vi "Teleop.vi"(10 "Match Info":T4={"Autonomous Elapsed Seconds"=0.0, "TeleOp Elapsed Seconds"=0.0, "Disabled Elapsed Seconds"=0.0, "Visited Autonomous"=FALSE, "Visited TeleOp"=FALSE, "Visited Disabled"=FALSE, "Autonomous Settings"={"Autonomous Style"=enum."Independent", "VI Refnum"=refnum}}, 11 "Call Context":T5) -> ()   [LabVIEW 2013]
doc: "This VI is called for each TeleOp packet received from the DS where the robot is not disabled. It is often used to read from the joysticks and update I/O or to update setpoints for timed control loops. It should complete and return within 20 milliseconds or it may miss DS packets."
uses:
  <vilib>/Rock Robotics/WPI/DriverStation/WPI_DriverStationDerivedRobotMode.ctl
  <vilib>/Rock Robotics/WPI/DriverStation/WPI_DriverStationMatch Info.ctl
  <vilib>/Rock Robotics/WPI/Solenoid/WPI_SolenoidValue.ctl
  <vilib>/Rock Robotics/WPI/Relay/WPI_RelayValue.ctl
  Robot Global Data.vi
  <vilib>/Rock Robotics/Network Tables/SD Read Number.vi
  <vilib>/Rock Robotics/WPI/Solenoid/WPI_SolenoidGetEnum.vi
  <vilib>/Rock Robotics/WPI/Compressor/WPI_CompressorGetSetRefNum.vi
  <vilib>/Rock Robotics/WPI/Solenoid/WPI_SolenoidSetEnum.vi
  <vilib>/Rock Robotics/WPI/Joystick/WPI_JoystickGetSetRefNum.vi
  <vilib>/Rock Robotics/WPI/RobotDrive/WPI_RobotDriveGetSetRefNum.vi
panel:
  in  "Grabber Timer":dbl
  in  "GrabberCurrentTarget":dbl
  in  "HasGrabberBeenReset":bool
  in  "ToughBoxEncoderTopPosition":dbl
  in  "Current Grabber Status":T1(ring)
  out "Waveform Chart 2":dbl(graph)
  in  "Run Grabber PID 2":bool
  out "Reed Switch 2":bool
  out "Reed Switch 1":bool
  out "Top Limit Tripped":bool
  out "Micro Switch":bool
  out "Bottom Limit Tripped":bool
  out "Axis Value  6":dbl
  out "Axis Value 5":dbl
  out "Axis Value 4":dbl
  in  "Grabber Axis Value":T2(ring)
  in  "Current Shooter Status":T3(ring)
  out "Waveform Chart":dbl(graph)
  out "Mechanism Moving Up":bool
  out "Mechanism Moving Down":bool
  out "Time Since Button Pressed":dbl
  in  "Manual Override Activated":bool
  in  "Button 2 Pressed":bool
  in  "Firing Pin Forward":bool
  in  "Mechanism Piston Forward":bool
  in  "Tick Taken":bool
  out "Time at Gather":dbl
  out "Timer for firing mech":dbl
  in  "Mechanism Status":string
types:
  T1 = enum16{"Resetting", "Going Up", "Going Up Slow", "In Shooting Position", "Going Down", "Going Down Slow", "In Loading Position"}
  T2 = enum16{"Less Than Zero", "Greater Than Zero", "Equal To Zero"}
  T3 = enum16{"Retracting", "Firing", "Ready to fire", "Pulling back", "Just fired"}
  T4 = typedef "WPI_DriverStationMatch Info.ctl" = cluster{"Autonomous Elapsed Seconds":dbl, "TeleOp Elapsed Seconds":dbl, "Disabled Elapsed Seconds":dbl, "Visited Autonomous":bool, "Visited TeleOp":bool, "Visited Disabled":bool, "Autonomous Settings":cluster{"Autonomous Style":enum16{"Iterative", "Independent"}, "VI Refnum":refnum<vi>}}
  T5 = typedef "WPI_DriverStationDerivedRobotMode.ctl" = enum16{"Init", "Execute", "Stop"}
  T6 = typedef "WPI_SolenoidValue.ctl" = enum16{"Off", "On", "Forward", "Reverse"}
  T7 = enum16{"Resetting", "Going Up", "Going Up Slow", "In Shooting Position", "Going Down", "Going Down Slow", "In Loading Position", ""}
  T8 = typedef "WPI_DigitalInputDevRef.ctl" = cluster{"DevStatus":errorcluster, "DIO Channel":T9, "Digital Module":T10}
  T9 = typedef "FPGA_DIOChannel.ctl" = enum8{"DIO 1", "DIO 2", "DIO 3", "DIO 4", "DIO 5", "DIO 6", "DIO 7", "DIO 8", "DIO 9", "DIO 10", "DIO 11", "DIO 12", "DIO 13", "DIO 14", "Invalid"}
  T10 = typedef "FPGA_TypedefDigitalModule.ctl" = enum16{"Digital Module 1", "Digital Module 2"}
  T11 = typedef "WPI_MotorControlDeviceRef.ctl" = cluster{"DeviceStatus":errorcluster, "Type":enum16{"PWM", "CAN"}, "PWM":cluster{"Digital Module":T10, "PWM Channel":T12, "DeadBand":T13}, "CAN":cluster{"Device Number":u8, "Control Mode":T14, "Semaphore":T15, "Max Vout":dbl}, "Invert":bool, "TransformRef":T16, "InvTransformRef":T16}
  T12 = typedef "FPGA_DIOPWMChannel.ctl" = enum8{"PWM 1", "PWM 2", "PWM 3", "PWM 4", "PWM 5", "PWM 6", "PWM 7", "PWM 8", "PWM 9", "PWM 10", "Invalid"}
  T13 = typedef "WPI_PWMDeadband.ctl" = cluster{"Name":string, "maxPositivePwm":i32, "minPositivePwm":i32, "centerPwm":i32, "maxNegativePwm":i32, "minNegativePwm":i32, "angularRange":u16}
  T14 = typedef "WPI_CANJaguar_ControlMode.ctl" = enum8{"Percent VBus", "Current", "Speed", "Position", "Voltage"}
  T15 = typedef "Semaphore RefNum" = refnum<k1>
  T16 = typedef "WPI_PWMTransform_ConPane.ctl" = refnum<vi>
  T17 = typedef "WPI_SolenoidDevRef.ctl" = cluster{"DevStatus":errorcluster, "Solenoid Module":T18, "Forward Solenoid Channel":T19, "Reverse Solenoid Channel":T19}
  T18 = typedef "FPGA_TypedefSolenoidModule.ctl" = enum16{"Solenoid Module 1", "Solenoid Module 2"}
  T19 = typedef "WPI_SolenoidChannel.ctl" = enum8{"Solenoid 1", "Solenoid 2", "Solenoid 3", "Solenoid 4", "Solenoid 5", "Solenoid 6", "Solenoid 7", "Solenoid 8", "Invalid"}
  T20 = typedef "WPI_JoystickDevRef.ctl" = cluster{"Device":T21}
  T21 = typedef "WPI_JoystickDeviceEnum.ctl" = enum16{"USB 1", "USB 2", "USB 3", "USB 4", "Kinect 1", "Kinect 2"}
  T22 = typedef "WPI_JoystickButtonState.ctl" = cluster{"Button 1":bool, "Button 2":bool, "Button 3":bool, "Button 4":bool, "Button 5":bool, "Button 6":bool, "Button 7":bool, "Button 8":bool, "Button 9":bool, "Button 10":bool, "Button 11":bool, "Button 12":bool}
  T23 = typedef "WPI_EncoderDevRef.ctl" = cluster{"DevStatus":errorcluster, "EncoderIndex":T24, "CounterIndex":T25, "DistancePerCount":dbl, "Decoding Type":T26}
  T24 = typedef "FPGA_EncoderIdx.ctl" = enum8{"Enc 0", "Enc 1", "Enc 2", "Enc 3", "Invalid"}
  T25 = typedef "FPGA_CounterCtrSystemIndex.ctl" = enum8{"Ctr 0", "Ctr 1", "Ctr 2", "Ctr 3", "Ctr 4", "Ctr 5", "Ctr 6", "Ctr 7", "Invalid"}
  T26 = typedef "WPI_EncoderType.ctl" = enum16{"1x", "2x", "4x"}
  T27 = typedef "WPI_RelayDevRef.ctl" = cluster{"DevStatus":errorcluster, "Relay Channel":T28, "Digital Module":T10, "Relay Direction":T29}
  T28 = typedef "FPGA_DIORelayChannel.ctl" = enum8{"Relay 1", "Relay 2", "Relay 3", "Relay 4", "Relay 5", "Relay 6", "Relay 7", "Relay 8", "Invalid"}
  T29 = typedef "WPI_RelayDirection.ctl" = enum16{"Both directions", "Forward only", "Reverse only"}
  T30 = typedef "WPI_CompressorDevRef.ctl" = cluster{"DevStatus":errorcluster, "DigitalInputDevRef":T8, "RelayDevRef":T27}
  T31 = typedef "WPI_RelayValue.ctl" = enum16{"Off", "On", "Forward", "Reverse"}
  T32 = typedef "WPI_AnalogChannelDevRef.ctl" = cluster{"DevStatus":errorcluster, "Analog Module":T33, "Analog Channel":T34}
  T33 = typedef "FPGA_TypedefAnalogModule.ctl" = enum16{"Analog Module 1", "Analog Module 2"}
  T34 = typedef "FPGA_AIChannel.ctl" = enum8{"AI 1", "AI 2", "AI 3", "AI 4", "AI 5", "AI 6", "AI 7", "AI 8", "Invalid"}
  T35 = typedef "WPI_ServoDeviceRef.ctl" = cluster{"DeviceStatus":errorcluster, "Digital Module":T10, "PWM Channel":T12, "DeadBand":T13}
  T36 = cluster{"axis 1 (x)":dbl, "axis 2 (y)":dbl, "axis 3 (throttle)":dbl, "axis 4":dbl, "axis 5":dbl, "axis 6":dbl}
  T37 = typedef "WPI_RobotDriveDevRef.ctl" = cluster{"DevStatus":errorcluster, "Motors[]":T11[], "Square Inputs":bool, "Max Output":dbl, "Isochronous":bool}
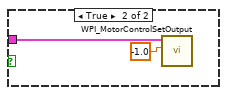
[diagram p3: hidden frame]
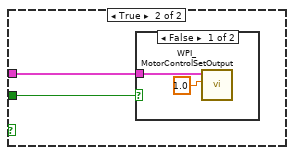
[diagram p4: hidden frame]
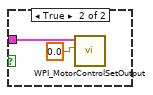
[diagram p5: hidden frame]
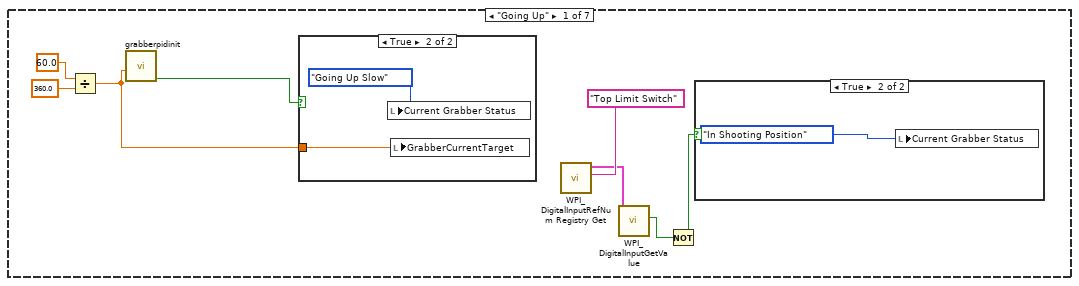
[diagram p7: hidden frame]
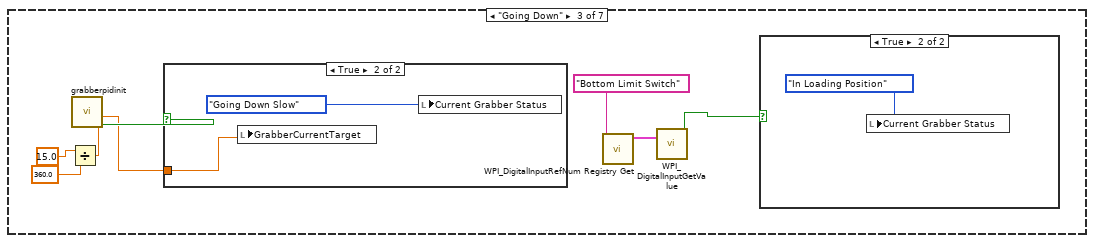
[diagram p11: hidden frame]
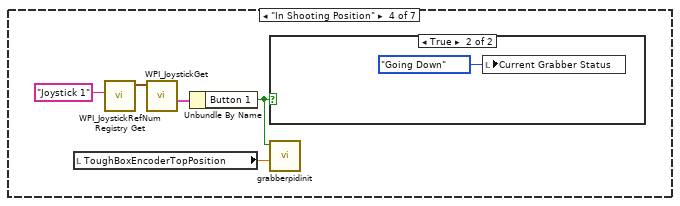
[diagram p14: hidden frame]
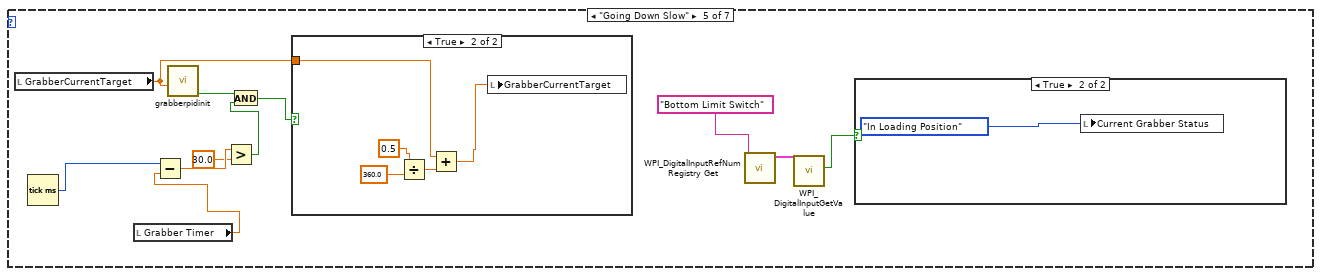
[diagram p16: hidden frame]
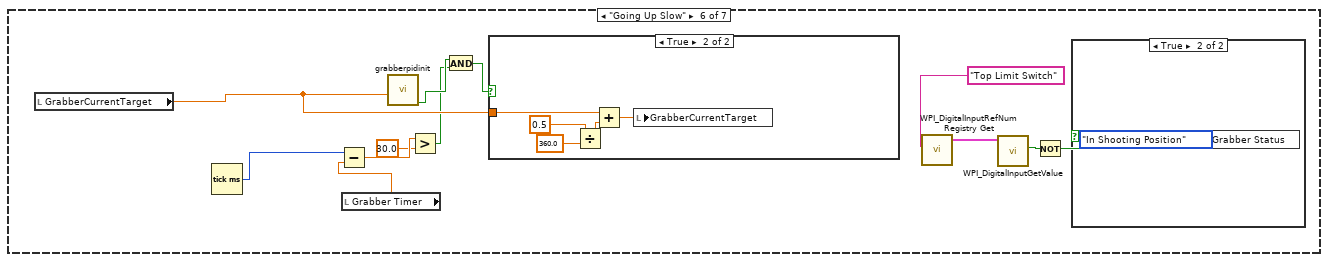
[diagram p19: hidden frame]
diagram:
  (unwired) "Below code is for running the Raising/Lowering motors"
  (unwired) "This code sets the toggle rate used by the Periodic Tasks VI.  For teleop mode we flash the USER1 LED on the cRIO at a fast rate.  Look at the Periodic Tasks VI to see how this global value is used."
  (unwired) "This VI is called each time a TeleOp DS packet is received.  Use it to respond to new joystick or Driver Station values.\n\nCommon tasks include reading the joysticks and updating motors, and updating setpoints for periodic loops.\n\nYou can open I/O on the FIRST Call, or in the Begin.vi."
  # "one encoder"
  # "Check me!"
  # "If no buttons pressed - 0\nIf left pressed = 7\nIf right pressed = -7\nIf both = 0"
  # "Publish the Robot Drive Motor\nvalues to the dashboard"
  # "Publish the joystick data the\nrobot sees to the dashboard"
  # "Each time we enter, report that\nwe are running teleop"
  # "Use to differentiate between\nFirst, Last, and Intermediate calls"
  # "Read Joystick X and Y values and update motor values"
  n1 = call <vilib>:"SD Read Boolean.vi"("Name"="Manual Mechanism Override") -> ("Boolean"=w7:bool)  [unwired: 8 in, 2 out]
  n2 = Not(x=w7) -> (.not. x?=w8:bool)
  n3 = case shown="True" w8 {
    frame False {
    }
    frame True {
      n4 = local read "Current Grabber Status"() -> (w131:T1)
      n5 = case shown="\"In Loading Position\"" w131 {
        frame "Going Up" {
          n6 = Divide(x=60.0 ("setpoint"), y=360.0) -> (x/y=w132:dbl)
          n7 = call "grabberpidinit.vi"("setpoint"=w132) -> ("Done? 2"=w139:bool)  [unwired: 10 in]
          n8 = case shown="True" w139 {
            tunnel: w132 -> [_ w141]
            frame False {
            }
            frame True {
              n9 = local write "Current Grabber Status"(T1."Going Up Slow" ("Current Grabber Status")) -> ()
              n10 = local write "GrabberCurrentTarget"(w141) -> ()
            }
          }
          n11 = call <vilib>:"WPI_DigitalInputRefNum Registry Get.vi"("refnum name"="Top Limit Switch") -> ("DigitalInputDevRef"=w137:T8)  [unwired: 9 in, 1 out]
          n12 = call <vilib>:"WPI_DigitalInputGetValue.vi"("DigitalInputDevRef"=w137) -> ("Value"=w136:bool)  [unwired: 8 in, 2 out]
          n13 = Not(x=w136) -> (.not. x?=w135:bool)
          n14 = case shown="True" w135 {
            frame False {
            }
            frame True {
              n15 = local write "Current Grabber Status"(T1."In Shooting Position" ("Current Grabber Status")) -> ()
            }
          }
        }
        frame "In Loading Position" {
          # "Change to the UltraSonic Sensor\nwhen possible"
          n16 = call "grabberpidinit.vi"("setpoint"=0.0) -> ("Done? 2"=w143:bool)  [unwired: 10 in]
          n17 = call <vilib>:"WPI_MotorControlRefNum Registry Get.vi"("refnum name"="Snowblower") -> ("MotorControlDevRef"=w155:T11)  [unwired: 9 in, 1 out]
          n18 = call <vilib>:"WPI_MotorControlSetOutput.vi"("Output"=-1.0, "MotorControlDevRef"=w155) -> ()  [unwired: 7 in, 3 out]
          n19 = call <vilib>:"WPI_SolenoidRefNum Registry Get.vi"("refnum name"="Grabber Pistons Solenoid") -> ("error out"=w152:errorcluster, "SolenoidDevRef"=w151:T17)  [unwired: 9 in]
          n20 = call-poly <vilib>:"WPI_SolenoidSet.vi"("error in (no error)"=w152, "Value"=WPI_SolenoidValue."Reverse", "SolenoidDevRef"=w151) -> ()  [unwired: 7 in, 2 out]
          n21 = call <vilib>:"WPI_JoystickRefNum Registry Get.vi"("refnum name"="Joystick 1") -> ("JoystickDevRef"=w147:T20)  [unwired: 1 in, 9 out]
          n22 = call <vilib>:"WPI_JoystickGet.vi"("JoystickDevRef"=w147) -> ("Buttons"=w146:T22)  [unwired: 1 in, 5 out]
          n23 = Unbundle By Name(w146) -> ("Button 4"=w144:bool)
          n24 = And(x=w143, y=w144) -> (x .and. y?=w145:bool)
          n25 = case shown="True" w145 {
            frame False {
            }
            frame True {
              n26 = local write "Current Grabber Status"(T1."Going Up" ("Current Grabber Status")) -> ()
            }
          }
        }
        frame "Going Down" {
          n27 = Divide(x=15.0, y=360.0) -> (x/y=w158:dbl)
          n28 = call "grabberpidinit.vi"("setpoint"=w158) -> ("Done? 2"=w164:bool)  [unwired: 10 in]
          n29 = case shown="True" w164 {
            tunnel: w158 -> [_ w166]
            frame False {
            }
            frame True {
              n30 = local write "GrabberCurrentTarget"(w166) -> ()
              n31 = local write "Current Grabber Status"(T1."Going Down Slow" ("Current Grabber Status")) -> ()
            }
          }
          n32 = call <vilib>:"WPI_DigitalInputRefNum Registry Get.vi"("refnum name"="Bottom Limit Switch") -> ("DigitalInputDevRef"=w162:T8)  [unwired: 9 in, 1 out]
          n33 = call <vilib>:"WPI_DigitalInputGetValue.vi"("DigitalInputDevRef"=w162) -> ("Value"=w161:bool)  [unwired: 8 in, 2 out]
          n34 = case shown="True" w161 {
            frame False {
            }
            frame True {
              n35 = local write "Current Grabber Status"(T1."In Loading Position" ("Current Grabber Status")) -> ()
            }
          }
        }
        frame "In Shooting Position" {
          n36 = local read "ToughBoxEncoderTopPosition"() -> (w169:dbl)
          n37 = call <vilib>:"WPI_JoystickRefNum Registry Get.vi"("refnum name"="Joystick 1") -> ("JoystickDevRef"=w171:T20)  [unwired: 1 in, 9 out]
          n38 = call <vilib>:"WPI_JoystickGet.vi"("JoystickDevRef"=w171) -> ("Buttons"=w170:T22)  [unwired: 1 in, 5 out]
          n39 = Unbundle By Name(w170) -> ("Button 1"=w168:bool)
          n40 = case shown="True" w168 {
            frame False {
            }
            frame True {
              n41 = local write "Current Grabber Status"(T7."Going Down" ("Current Grabber Status")) -> ()
            }
          }
          n42 = call "grabberpidinit.vi"("setpoint"=w169, "reinitialize? (F) 2"=w168) -> ()  [unwired: 9 in, 1 out]
        }
        frame "Going Down Slow" {
          n43 = local read "GrabberCurrentTarget"() -> (w174:dbl)
          n44 = Tick Count (ms)() -> (millisecond timer value=w184:u32)
          n45 = local read "Grabber Timer"() -> (w181:dbl)
          n46 = Subtract(x=w184, y=w181) -> (x-y=w183:dbl)
          n47 = call "grabberpidinit.vi"("setpoint"=w174) -> ("Done? 2"=w180:bool)  [unwired: 10 in]
          n48 = Greater?(x=w183, y=30.0) -> (0:w179:bool)
          n49 = And(x=w180, y=w179) -> (x .and. y?=w178:bool)
          n50 = case shown="True" w178 {
            tunnel: w174 -> [_ w187]
            frame False {
            }
            frame True {
              n51 = Divide(x=0.5, y=360.0) -> (x/y=w188:dbl)
              n52 = Add(x=w187, y=w188) -> (x+y=w186:dbl)
              n53 = local write "GrabberCurrentTarget"(w186) -> ()
            }
          }
          n54 = call <vilib>:"WPI_DigitalInputRefNum Registry Get.vi"("refnum name"="Bottom Limit Switch") -> ("DigitalInputDevRef"=w176:T8)  [unwired: 9 in, 1 out]
          n55 = call <vilib>:"WPI_DigitalInputGetValue.vi"("DigitalInputDevRef"=w176) -> ("Value"=w175:bool)  [unwired: 8 in, 2 out]
          n56 = case shown="True" w175 {
            frame False {
            }
            frame True {
              n57 = local write "Current Grabber Status"(T1."In Loading Position" ("Current Grabber Status")) -> ()
            }
          }
        }
        frame "Going Up Slow" {
          n58 = local read "GrabberCurrentTarget"() -> (w202:dbl)
          n59 = Tick Count (ms)() -> (millisecond timer value=w201:u32)
          n60 = local read "Grabber Timer"() -> (w200:dbl)
          n61 = Subtract(x=w201, y=w200) -> (x-y=w199:dbl)
          n62 = call "grabberpidinit.vi"("setpoint"=w202) -> ("Done? 2"=w197:bool)  [unwired: 10 in]
          n63 = Greater?(x=w199, y=30.0) -> (0:w196:bool)
          n64 = And(x=w197, y=w196) -> (x .and. y?=w195:bool)
          n65 = case shown="True" w195 {
            tunnel: w202 -> [_ w207]
            frame False {
            }
            frame True {
              n66 = Divide(x=0.5 ("y"), y=360.0) -> (x/y=w204:dbl)
              n67 = Add(x=w207, y=w204) -> (x+y=w208:dbl)
              n68 = local write "GrabberCurrentTarget"(w208) -> ()
            }
          }
          n69 = call <vilib>:"WPI_DigitalInputRefNum Registry Get.vi"("refnum name"="Top Limit Switch") -> ("DigitalInputDevRef"=w192:T8)  [unwired: 9 in, 1 out]
          n70 = call <vilib>:"WPI_DigitalInputGetValue.vi"("DigitalInputDevRef"=w192) -> ("Value"=w194:bool)  [unwired: 8 in, 2 out]
          n71 = Not(x=w194) -> (.not. x?=w193:bool)
          n72 = case shown="True" w193 {
            frame False {
            }
            frame True {
              n73 = local write "Current Grabber Status"(T1."In Shooting Position" ("Current Grabber Status")) -> ()
            }
          }
        }
        frame "Resetting", Default {
          n74 = local read "GrabberCurrentTarget"() -> (w221:dbl)
          n75 = call <vilib>:"WPI_DigitalInputRefNum Registry Get.vi"("refnum name"="Bottom Limit Switch") -> ("DigitalInputDevRef"=w211:T8)  [unwired: 9 in, 1 out]
          n76 = Equal?(x=w221, y=0.0) -> (x = y?=w220:bool)
          n77 = call <vilib>:"WPI_DigitalInputGetValue.vi"("DigitalInputDevRef"=w211) -> ("Value"=w209:bool)  [unwired: 8 in, 2 out]
          n78 = case shown="True" w220 {
            tunnel: [w233 w234] -> w219
            tunnel: w221 -> [w233 _]
            frame False {
            }
            frame True {
              # "one encoder"
              n79 = call <vilib>:"WPI_EncoderRefNum Registry Get.vi"("refnum name"="Tough Box Encoder") -> ("error out"=w237:errorcluster, "EncoderDevRef"=w236:T23)  [unwired: 9 in]
              n80 = call <vilib>:"WPI_EncoderGet.vi"("error in (no error)"=w237, "EncoderDevRef"=w236) -> ("Distance"=w234:dbl)  [unwired: 4 in, 5 out]
              n81 = local write "GrabberCurrentTarget"(w234) -> ()
            }
          }
          n82 = case shown="True" w209 {
            frame False {
            }
            frame True {
              n83 = call <vilib>:"WPI_EncoderRefNum Registry Get.vi"("refnum name"="Tough Box Encoder") -> ("error out"=w225:errorcluster, "EncoderDevRef"=w224:T23)  [unwired: 9 in]
              n84 = local write "Current Grabber Status"(T7."In Loading Position" ("Current Grabber Status")) -> ()
              n85 = call <vilib>:"WPI_EncoderReset.vi"("error in (no error)"=w225, "EncoderDevRef"=w224) -> ()  [unwired: 8 in, 2 out]
            }
          }
          n86 = local read "Grabber Timer"() -> (w217:dbl)
          n87 = Tick Count (ms)() -> (millisecond timer value=w218:u32)
          n88 = Subtract(x=w218, y=w217) -> (x-y=w216:dbl)
          n89 = call "grabberpidinit.vi"("setpoint"=w219, "reinitialize? (F) 2"=w209) -> ("Done? 2"=w212:bool)  [unwired: 9 in]
          n90 = Greater?(x=w216, y=30.0) -> (0:w213:bool)
          n91 = And(x=w212, y=w213) -> (x .and. y?=w214:bool)
          n92 = case shown="True" w214 {
            tunnel: w219 -> [_ w229]
            frame False {
            }
            frame True {
              n93 = Tick Count (ms)() -> (millisecond timer value=w227:u32)
              n94 = Divide(x=0.5, y=360.0) -> (x/y=w232:dbl)
              n95 = Subtract(x=w229, y=w232) -> (x-y=w228:dbl)
              n96 = local write "Grabber Timer"(w227) -> ()
              n97 = local write "GrabberCurrentTarget"(w228) -> ()
            }
          }
        }
      }
    }
  }
  n98 = local write "Mechanism Piston Forward"(FALSE) -> ()
  n99 = local write "Firing Pin Forward"(FALSE) -> ()
  n100 = call <vilib>:"WPI_DriverStationReport Robot Code State.vi"("TeleOp"=TRUE ("Autonomous")) -> ()  [unwired: 10 in, 1 out]
  n101 = global write "Robot Global Data.vi" "LED toggle rate (ms)"(u32 100 ("LED ms toggle rate")) -> ()
  n102 = call <vilib>:"WPI_JoystickRefNum Registry Get.vi"("refnum name"="Joystick 1") -> ("JoystickDevRef"=w109:T20)  [unwired: 1 in, 9 out]
  n103 = Unbundle By Name("Match Info") -> ()  [unwired: 1 out]
  n104 = call <vilib>:"SD Read Boolean.vi"("Name"="Light Ring On") -> ("Boolean"=w19:bool)  [unwired: 8 in, 2 out]
  n105 = call <vilib>:"WPI_RelayRefNum Registry Get.vi"("refnum name"="Light Ring") -> ("RelayDevRef"=w18:T27)  [unwired: 9 in, 1 out]
  n106 = call <vilib>:"WPI_DigitalInputRefNum Registry Get.vi"("refnum name"="Reed Switch 1") -> ("DigitalInputDevRef"=w55:T8)  [unwired: 9 in, 1 out]
  n107 = call <vilib>:"WPI_DigitalInputRefNum Registry Get.vi"("refnum name"="Reed Switch 2") -> ("DigitalInputDevRef"=w48:T8)  [unwired: 9 in, 1 out]
  n108 = call <vilib>:"WPI_DigitalInputRefNum Registry Get.vi"("refnum name"="Reed Switch 2") -> ("DigitalInputDevRef"=w52:T8)  [unwired: 9 in, 1 out]
  n109 = call <vilib>:"WPI_DigitalInputRefNum Registry Get.vi"("refnum name"="Micro Switch 1") -> ("DigitalInputDevRef"=w68:T8)  [unwired: 9 in, 1 out]
  n110 = call <vilib>:"WPI_DigitalInputRefNum Registry Get.vi"("refnum name"="Micro Switch 1") -> ("DigitalInputDevRef"=w44:T8)  [unwired: 9 in, 1 out]
  n111 = call <vilib>:"WPI_DigitalInputRefNum Registry Get.vi"("refnum name"="Top Limit Switch") -> ("DigitalInputDevRef"=w61:T8)  [unwired: 9 in, 1 out]
  n112 = call <vilib>:"WPI_JoystickGet.vi"("JoystickDevRef"=w109) -> ("Buttons"=w108:T22)  [unwired: 1 in, 5 out]
  n113 = call <vilib>:"SD Read Boolean.vi"("Name"="Compressor On/Off") -> ("Boolean"=w70:bool)  [unwired: 8 in, 2 out]
  n114 = call <vilib>:"WPI_CompressorRefNum Registry Get.vi"("refnum name"="Compressor") -> ("CompressorDevRef"=w71:T30)  [unwired: 9 in, 1 out]
  n115 = call <vilib>:"WPI_DigitalInputRefNum Registry Get.vi"("refnum name"="Bottom Limit Switch") -> ("DigitalInputDevRef"=w76:T8)  [unwired: 9 in, 1 out]
  n116 = call <vilib>:"WPI_DigitalInputGetValue.vi"("DigitalInputDevRef"=w55) -> ("Value"=→"Reed Switch 1":bool)  [unwired: 8 in, 2 out]
  n117 = call <vilib>:"WPI_DigitalInputGetValue.vi"("DigitalInputDevRef"=w48) -> ("Value"=w47:bool)  [unwired: 8 in, 2 out]
  n118 = call <vilib>:"WPI_DigitalInputGetValue.vi"("DigitalInputDevRef"=w52) -> ("Value"=→"Reed Switch 2":bool)  [unwired: 8 in, 2 out]
  n119 = call <vilib>:"WPI_DigitalInputGetValue.vi"("DigitalInputDevRef"=w68) -> ("Value"=→"Micro Switch":bool)  [unwired: 8 in, 2 out]
  n120 = call <vilib>:"WPI_DigitalInputGetValue.vi"("DigitalInputDevRef"=w44) -> ("Value"=w43:bool)  [unwired: 8 in, 2 out]
  n121 = case shown="True" w19 {
    tunnel: w18 -> [w238 w241]
    frame False {
      n122 = call <vilib>:"WPI_RelaySet.vi"("RelayValue"=WPI_RelayValue."Off", "RelayDevRef"=w238) -> ()  [unwired: 8 in, 2 out]
    }
    frame True {
      n123 = call <vilib>:"WPI_RelaySet.vi"("RelayValue"=WPI_RelayValue."Forward", "RelayDevRef"=w241) -> ()  [unwired: 8 in, 2 out]
    }
  }
  n124 = call <vilib>:"WPI_DigitalInputGetValue.vi"("DigitalInputDevRef"=w61) -> ("Value"=→"Top Limit Tripped":bool)  [unwired: 8 in, 2 out]
  n125 = call <vilib>:"SD Read Boolean.vi"("Name"="Manual Mechanism Override") -> ("Boolean"=w1:bool)  [unwired: 8 in, 2 out]
  n126 = call <vilib>:"WPI_AnalogChannelRefNum Registry Get.vi"("refnum name"="Grabber Ultrasonic Sensor") -> ("AIDeviceRef"=w16:T32)  [unwired: 9 in, 1 out]
  n127 = Unbundle By Name(w108) -> ("Button 8"=w107:bool)
  n128 = case shown="False" w70 {
    tunnel: w71 -> [w242 w243]
    frame False {
      n129 = call <vilib>:"WPI_CompressorStop.vi"("CompressorDevRef"=w242) -> ()  [unwired: 9 in, 2 out]
    }
    frame True {
      n130 = call <vilib>:"WPI_CompressorStart.vi"("CompressorDevRef"=w243) -> ()  [unwired: 9 in, 2 out]
    }
  }
  n131 = call <vilib>:"WPI_DigitalInputGetValue.vi"("DigitalInputDevRef"=w76) -> ("Value"=→"Bottom Limit Tripped":bool)  [unwired: 8 in, 2 out]
  n132 = Not(x=w47) -> (.not. x?=w46:bool)
  n133 = call-poly <vilib>:"SD Read Value.vi"("Name"="Camera Pitch Control") -> ("Numeric"=w91:dbl)  [unwired: 8 in, 2 out]
  n134 = call <vilib>:"WPI_SolenoidRefNum Registry Get.vi"("refnum name"="Grabber Pistons Solenoid") -> ("SolenoidDevRef"=w79:T17)  [unwired: 9 in, 1 out]
  n135 = call <vilib>:"SD Read Boolean.vi"("Name"="Manual Mechanism Override") -> ("Boolean"=w56:bool)  [unwired: 8 in, 2 out]
  n136 = call <vilib>:"WPI_SolenoidRefNum Registry Get.vi"("refnum name"="Drawback Pistons") -> ("SolenoidDevRef"=w100:T17)  [unwired: 9 in, 1 out]
  n137 = call <vilib>:"WPI_SolenoidRefNum Registry Get.vi"("refnum name"="Firing Pin Solenoid") -> ("SolenoidDevRef"=w102:T17)  [unwired: 9 in, 1 out]
  n138 = Not(x=w43) -> (.not. x?=w42:bool)
  n139 = call <vilib>:"WPI_ServoRefNum Registry Get.vi"("refnum name"="Camera Pitch Servo") -> ("ServoDeviceRef"=w92:T35)  [unwired: 9 in, 1 out]
  n140 = call-poly <vilib>:"SD Read Value.vi"("Name"="Camera Rotation Control") -> ("Numeric"=w95:dbl)  [unwired: 8 in, 2 out]
  n141 = call <vilib>:"WPI_AnalogChannelGetVoltage.vi"("AIDeviceRef"=w16) -> ("Voltage"=→"Waveform Chart":dbl)  [unwired: 8 in, 2 out]
  n142 = call <vilib>:"WPI_ServoRefNum Registry Get.vi"("refnum name"="Camera Rotation Servo") -> ("ServoDeviceRef"=w94:T35)  [unwired: 9 in, 1 out]
  n143 = call <vilib>:"SD Write Boolean.vi"("Boolean"=w46, "Name"="Are Drawback Pistons Extended") -> ()  [unwired: 8 in, 2 out]
  n144 = call <vilib>:"SD Write Boolean.vi"("Boolean"=w42, "Name"="Is The Firing Pin Piston Extended") -> ()  [unwired: 8 in, 2 out]
  n145 = call <vilib>:"SD Read Boolean.vi"("Name"="Manual Mechanism Override") -> ("Boolean"=w85:bool)  [unwired: 8 in, 2 out]
  n146 = call-poly <vilib>:"WPI_SolenoidGet.vi"("SolenoidDevRef"=w79) -> ("Value"=w81:T6)  [unwired: 8 in, 2 out]
  n147 = call <vilib>:"WPI_JoystickRefNum Registry Get.vi"("refnum name"="Joystick 1") -> ("JoystickDevRef"=w114:T20)  [unwired: 1 in, 9 out]
  n148 = call <vilib>:"WPI_ServoSetAngle.vi"("Angle"=w91, "ServoDeviceRef"=w92) -> ()  [unwired: 8 in, 2 out]
  n149 = call <vilib>:"WPI_ServoSetAngle.vi"("Angle"=w95, "ServoDeviceRef"=w94) -> ()  [unwired: 8 in, 2 out]
  n150 = Equal?(x=w81, y=WPI_SolenoidValue."Forward") -> (x = y?=w14:bool)
  n151 = case shown="True" w56 {
    tunnel: w102 -> [_ w262]
    tunnel: w100 -> [_ w261]
    tunnel: w79 -> [_ w244]
    frame False {
    }
    frame True {
      n152 = call <vilib>:"SD Read Boolean.vi"("Name"="Grabber Pistons Extended") -> ("Boolean"=w253:bool)  [unwired: 8 in, 2 out]
      n153 = call <vilib>:"SD Read Boolean.vi"("Name"="Drawback Pistons Activated") -> ("Boolean"=w245:bool)  [unwired: 8 in, 2 out]
      n154 = call <vilib>:"SD Read Boolean.vi"("Name"="Firing Pin Piston Extended") -> ("Boolean"=w259:bool)  [unwired: 8 in, 2 out]
      n155 = case shown="True" w245 {
        tunnel: w261 -> [_ w270]
        frame False {
        }
        frame True {
          n156 = call <vilib>:"SD Read Boolean.vi"("Name"="Drawback Piston Extended") -> ("Boolean"=w268:bool)  [unwired: 8 in, 2 out]
          n157 = Equal?(x=w268, y=FALSE) -> (x = y?=w266:bool)
          n158 = Select(t=WPI_SolenoidValue."Forward" ("Value"), s=w266, f=WPI_SolenoidValue."Reverse") -> (s? t:f=w263:T6)
          n159 = call-poly <vilib>:"WPI_SolenoidSet.vi"("Value"=w263, "SolenoidDevRef"=w270) -> ()  [unwired: 8 in, 2 out]
        }
      }
      n160 = Equal?(x=w253, y=FALSE) -> (x = y?=w251:bool)
      n161 = Equal?(x=w259, y=FALSE) -> (x = y?=w255:bool)
      n162 = Select(t=WPI_SolenoidValue."Forward" ("Value"), s=w251, f=WPI_SolenoidValue."Reverse") -> (s? t:f=w248:T6)
      n163 = Select(t=WPI_SolenoidValue."Forward" ("Value"), s=w255, f=WPI_SolenoidValue."Reverse") -> (s? t:f=w256:T6)
      n164 = call-poly <vilib>:"WPI_SolenoidSet.vi"("Value"=w248, "SolenoidDevRef"=w244) -> ()  [unwired: 8 in, 2 out]
      n165 = call-poly <vilib>:"WPI_SolenoidSet.vi"("Value"=w256, "SolenoidDevRef"=w262) -> ()  [unwired: 8 in, 2 out]
    }
  }
  n166 = Not(x=w14) -> (.not. x?=w13:bool)
  n167 = case shown="True" w107 {
    frame False {
    }
    frame True {
      n168 = global read "Robot Global Data.vi" "Time since  button 8 pressed"() -> (w271:dbl)
      n169 = Tick Count (ms)() -> (millisecond timer value=w275:u32)
      n170 = Subtract(x=w275, y=w271) -> (x-y=w274:dbl)
      n171 = Greater?(x=w274, y=300) -> (0:w272:bool)
      n172 = case shown="True" w272 {
        frame False {
        }
        frame True {
          n173 = Tick Count (ms)() -> (millisecond timer value=w276:u32)
          n174 = local read "Manual Override Activated"() -> (w280:bool)
          n175 = global write "Robot Global Data.vi" "Time since  button 8 pressed"(w276) -> ()
          n176 = Select(t=FALSE, s=w280, f=TRUE) -> (s? t:f=w277:bool)
          n177 = local write "Manual Override Activated"(w277) -> ()
        }
      }
    }
  }
  n178 = call <vilib>:"SD Read Boolean.vi"("Name"="Drawback Pistons Activated") -> ("Boolean"=w65:bool)  [unwired: 8 in, 2 out]
  n179 = Not(x=w85) -> (.not. x?=w64:bool)
  n180 = call <vilib>:"WPI_JoystickGet.vi"("JoystickDevRef"=w114) -> ("Buttons"=w113:T22, "Axes"=w106:T36)  [unwired: 1 in, 4 out]
  n181 = call <vilib>:"SD Write Boolean.vi"("Boolean"=w13, "Name"="Are Grabber Pistons Extended") -> ()  [unwired: 8 in, 2 out]
  n182 = Unbundle By Name(w113) -> ("Button 1"=w84:bool, "Button 5"=w40:bool, "Button 6"=w41:bool)  [unwired: 2 out]
  n183 = case shown="True" w1 {
    tunnel: w41 -> [_ w283]
    tunnel: w40 -> [_ w282]
    frame False {
    }
    frame True {
      n184 = call <vilib>:"WPI_MotorControlRefNum Registry Get.vi"("refnum name"="Snowblower") -> ("MotorControlDevRef"=w281:T11)  [unwired: 9 in, 1 out]
      n185 = case shown="False" w283 {
        tunnel: w282 -> [w286 w292]
        tunnel: w281 -> [w285 w291]
        frame False {
          n186 = case shown="False" w286 {
            tunnel: w285 -> [w288 w290]
            frame False {
              n187 = call <vilib>:"WPI_MotorControlSetOutput.vi"("Output"=0.0, "MotorControlDevRef"=w288) -> ()  [unwired: 7 in, 3 out]
            }
            frame True {
              n188 = call <vilib>:"WPI_MotorControlSetOutput.vi"("Output"=-1.0, "MotorControlDevRef"=w290) -> ()  [unwired: 7 in, 3 out]
            }
          }
        }
        frame True {
          n189 = case shown="False" w292 {
            tunnel: w291 -> [w294 w296]
            frame False {
              n190 = call <vilib>:"WPI_MotorControlSetOutput.vi"("Output"=1.0, "MotorControlDevRef"=w294) -> ()  [unwired: 7 in, 3 out]
            }
            frame True {
              n191 = call <vilib>:"WPI_MotorControlSetOutput.vi"("Output"=0.0, "MotorControlDevRef"=w296) -> ()  [unwired: 7 in, 3 out]
            }
          }
        }
      }
    }
  }
  n192 = And(x=w64, y=w65) -> (x .and. y?=w63:bool)
  n193 = Unbundle By Name(w106) -> ("axis 4"=→"Axis Value 4":dbl, "axis 5"=w59:dbl, "axis 6"=→"Axis Value  6":dbl)
  "Axis Value 5" <- w59
  n194 = Negate(x=w59) -> (-x=w58:dbl)
  n195 = Multiply(x=w58, y=0.75) -> (x*y=w35:dbl)
  n196 = call <vilib>:"WPI_DigitalInputRefNum Registry Get.vi"("refnum name"="Micro Switch 1") -> ("DigitalInputDevRef"=w32:T8)  [unwired: 9 in, 1 out]
  n197 = call <vilib>:"WPI_EncoderRefNum Registry Get.vi"("refnum name"="Tough Box Encoder") -> ("error out"=w3:errorcluster, "EncoderDevRef"=w4:T23)  [unwired: 9 in]
  n198 = call <vilib>:"WPI_DigitalInputRefNum Registry Get.vi"("refnum name"="Bottom Limit Switch") -> ("DigitalInputDevRef"=w37:T8)  [unwired: 9 in, 1 out]
  n199 = call <vilib>:"WPI_DigitalInputRefNum Registry Get.vi"("refnum name"="Top Limit Switch") -> ("DigitalInputDevRef"=w27:T8)  [unwired: 9 in, 1 out]
  n200 = call <vilib>:"WPI_DigitalInputGetValue.vi"("DigitalInputDevRef"=w32) -> ("Value"=w33:bool)  [unwired: 8 in, 2 out]
  n201 = call <vilib>:"WPI_DigitalInputGetValue.vi"("DigitalInputDevRef"=w37) -> ("Value"=w12:bool)  [unwired: 8 in, 2 out]
  n202 = call <vilib>:"WPI_DigitalInputGetValue.vi"("DigitalInputDevRef"=w27) -> ("Value"=w29:bool)  [unwired: 8 in, 2 out]
  n203 = Not(x=w29) -> (.not. x?=w30:bool)
  n204 = Not(x=w33) -> (.not. x?=w11:bool)
  n205 = case shown="True" w63 {
    tunnel: w84 -> [_ w297]
    frame False {
    }
    frame True {
      n206 = case shown="\"Firing\"" "Current Shooter Status" {
        tunnel: w297 -> [_ w305 _ _ _]
        frame "Firing" {
          n207 = Tick Count (ms)() -> (millisecond timer value=w299:u32)
          n208 = local write "Timer for firing mech"(w299) -> ()
          n209 = local write "Current Shooter Status"(T3."Just fired" ("Current Shooter Status")) -> ()
          n210 = call <vilib>:"WPI_SolenoidRefNum Registry Get.vi"("refnum name"="Firing Pin Solenoid") -> ("error out"=w303:errorcluster, "SolenoidDevRef"=w302:T17)  [unwired: 9 in]
          n211 = call-poly <vilib>:"WPI_SolenoidSet.vi"("error in (no error)"=w303, "Value"=WPI_SolenoidValue."Reverse", "SolenoidDevRef"=w302) -> ()  [unwired: 7 in, 2 out]
        }
        frame "Ready to fire" {
          # "Button one is pressed, so fire"
          n212 = case shown="True" w305 {
            frame False {
            }
            frame True {
              n213 = local write "Current Shooter Status"(T3."Firing" ("Current Shooter Status")) -> ()
            }
          }
        }
        frame "Pulling back" {
          n214 = call <vilib>:"WPI_DigitalInputRefNum Registry Get.vi"("refnum name"="Reed Switch 2") -> ("error out"=w308:errorcluster, "DigitalInputDevRef"=w309:T8)  [unwired: 9 in]
          n215 = call <vilib>:"WPI_DigitalInputGetValue.vi"("error in (no error)"=w308, "DigitalInputDevRef"=w309) -> ("Value"=w307:bool)  [unwired: 7 in, 2 out]
          n216 = call <vilib>:"WPI_SolenoidRefNum Registry Get.vi"("refnum name"="Drawback Pistons") -> ("error out"=w313:errorcluster, "SolenoidDevRef"=w312:T17)  [unwired: 9 in]
          n217 = call <vilib>:"WPI_SolenoidRefNum Registry Get.vi"("refnum name"="Firing Pin Solenoid") -> ("error out"=w317:errorcluster, "SolenoidDevRef"=w316:T17)  [unwired: 9 in]
          n218 = call-poly <vilib>:"WPI_SolenoidSet.vi"("error in (no error)"=w313, "Value"=WPI_SolenoidValue."Forward", "SolenoidDevRef"=w312) -> ()  [unwired: 7 in, 2 out]
          n219 = case shown="True" w307 {
            frame False {
            }
            frame True {
              n220 = Tick Count (ms)() -> (millisecond timer value=w319:u32)
              n221 = local write "Timer for firing mech"(w319) -> ()
              n222 = local write "Current Shooter Status"(T3."Retracting" ("Current Shooter Status")) -> ()
            }
          }
          n223 = call-poly <vilib>:"WPI_SolenoidSet.vi"("error in (no error)"=w317, "Value"=WPI_SolenoidValue."Reverse", "SolenoidDevRef"=w316) -> ()  [unwired: 7 in, 2 out]
        }
        frame "Retracting" {
          n224 = local read "Timer for firing mech"() -> (w334:dbl)
          n225 = call <vilib>:"WPI_DigitalInputRefNum Registry Get.vi"("refnum name"="Reed Switch 1") -> ("error out"=w326:errorcluster, "DigitalInputDevRef"=w327:T8)  [unwired: 9 in]
          n226 = call <vilib>:"WPI_DigitalInputGetValue.vi"("error in (no error)"=w326, "DigitalInputDevRef"=w327) -> ("Value"=w322:bool)  [unwired: 7 in, 2 out]
          n227 = call <vilib>:"WPI_SolenoidRefNum Registry Get.vi"("refnum name"="Firing Pin Solenoid") -> ("error out"=w337:errorcluster, "SolenoidDevRef"=w336:T17)  [unwired: 9 in]
          n228 = call-poly <vilib>:"WPI_SolenoidSet.vi"("error in (no error)"=w337, "Value"=WPI_SolenoidValue."Forward", "SolenoidDevRef"=w336) -> ()  [unwired: 7 in, 2 out]
          n229 = Not(x=w322) -> (.not. x?=w321:bool)
          n230 = Tick Count (ms)() -> (millisecond timer value=w331:u32)
          n231 = case shown="True" w321 {
            frame False {
            }
            frame True {
              n232 = local write "Current Shooter Status"(T3."Ready to fire" ("Current Shooter Status")) -> ()
            }
          }
          n233 = Subtract(x=w331, y=w334) -> (x-y=w333:dbl)
          n234 = Greater Or Equal?(x=1000, y=w333) -> (x >= y?=w324:bool)
          n235 = call <vilib>:"WPI_SolenoidRefNum Registry Get.vi"("refnum name"="Drawback Pistons") -> ("SolenoidDevRef"=w329:T17)  [unwired: 9 in, 1 out]
          n236 = And(x=TRUE, y=w324) -> (x .and. y?=w325:bool)
          n237 = case shown="True" w325 {
            tunnel: w329 -> [_ w340]
            frame False {
            }
            frame True {
              n238 = call-poly <vilib>:"WPI_SolenoidSet.vi"("Value"=WPI_SolenoidValue."Reverse", "SolenoidDevRef"=w340) -> ()  [unwired: 8 in, 2 out]
            }
          }
        }
        frame "Just fired", Default {
          # "When MicroSwitch is \nadded, Change this \nto read from that"
          n239 = local read "Timer for firing mech"() -> (w352:dbl)
          n240 = call <vilib>:"WPI_SolenoidRefNum Registry Get.vi"("refnum name"="Firing Pin Solenoid") -> ("error out"=w347:errorcluster, "SolenoidDevRef"=w346:T17)  [unwired: 9 in]
          n241 = Tick Count (ms)() -> (millisecond timer value=w349:u32)
          n242 = call-poly <vilib>:"WPI_SolenoidSet.vi"("error in (no error)"=w347, "Value"=WPI_SolenoidValue."Reverse", "SolenoidDevRef"=w346) -> ()  [unwired: 7 in, 2 out]
          n243 = Subtract(x=w349, y=w352) -> (x-y=w351:dbl)
          n244 = Greater Or Equal?(x=3000, y=w351) -> (x >= y?=w344:bool)
          n245 = And(x=TRUE, y=w344) -> (x .and. y?=w343:bool)
          n246 = case shown="True" w343 {
            frame False {
            }
            frame True {
              n247 = local write "Current Shooter Status"(T3."Pulling back" ("Current Shooter Status")) -> ()
            }
          }
        }
      }
    }
  }
  n248 = call <vilib>:"WPI_EncoderGet.vi"("error in (no error)"=w3, "EncoderDevRef"=w4) -> ("Distance"=→"Waveform Chart 2":dbl)  [unwired: 4 in, 5 out]
  n249 = Less?(x=w35, y=-0.01) -> (x < y?=w36:bool)
  n250 = And(x=w12, y=w11) -> (x .and. y?=w10:bool)
  n251 = And(x=w30, y=w11) -> (x .and. y?=w25:bool)
  n252 = Greater?(x=w35, y=0.01) -> (0:w26:bool)
  n253 = And(x=w10, y=w36) -> (x .and. y?=w23:bool)
  n254 = And(x=w26, y=w25) -> (x .and. y?=w24:bool)
  n255 = Or(x=w23, y=w24) -> (x .or. y?=w22:bool)
  n256 = case shown="True" w22 {
    tunnel: w35 -> [_ w357]
    frame False {
      n257 = call <vilib>:"WPI_MotorControlRefNum Registry Get.vi"("refnum name"="Fisher Price") -> ("MotorControlDevRef"=w355:T11)  [unwired: 9 in, 1 out]
      n258 = call <vilib>:"WPI_MotorControlSetOutput.vi"("Output"=0.0, "MotorControlDevRef"=w355) -> ()  [unwired: 7 in, 3 out]
    }
    frame True {
      n259 = call <vilib>:"WPI_MotorControlRefNum Registry Get.vi"("refnum name"="Fisher Price") -> ("MotorControlDevRef"=w359:T11)  [unwired: 9 in, 1 out]
      n260 = call <vilib>:"WPI_MotorControlSetOutput.vi"("Output"=w357, "MotorControlDevRef"=w359) -> ()  [unwired: 7 in, 3 out]
    }
  }
  n261 = call <vilib>:"WPI_JoystickRefNum Registry Get.vi"("refnum name"="Joystick 1") -> ("JoystickDevRef"=w126:T20)  [unwired: 1 in, 9 out]
  n262 = call <vilib>:"WPI_JoystickGet.vi"("JoystickDevRef"=w126) -> ("Buttons"=w124:T22, "Axes"=w121:T36)  [unwired: 1 in, 4 out]
  n263 = Unbundle By Name(w121) -> ("axis 1 (x)"=w90:dbl, "axis 2 (y)"=w88:dbl)  [unwired: 1 out]
  n264 = Cluster To Array(cluster=w121) -> (array=w120:dbl[])
  n265 = Cluster To Array(cluster=w124) -> (array=w123:bool[])
  n266 = Negate(x=w90) -> (-x=w89:dbl)
  n267 = Negate(x=w88) -> (-x=w87:dbl)
  n268 = call <vilib>:"WPI_RobotDriveRefNum Registry Get.vi"("refnum name"="Left and Right Motors") -> ("RobotDriveDevRef"=w128:T37)  [unwired: 1 in, 9 out]
  n269 = call <vilib>:"SD Write Numeric Array.vi"("Numeric Array"=w120, "Name"="Joystick 1/Axes") -> ()  [unwired: 8 in, 2 out]
  n270 = call <vilib>:"SD Write Boolean Array.vi"("Boolean Array"=w123, "Name"="Joystick 1/Buttons") -> ()  [unwired: 8 in, 2 out]
  n271 = call <vilib>:"WPI_RobotDriveArcadeDrive_Standard(NoSaturation).vi"("Y axis value"=w87, "X axis value"=w89, "RobotDriveDevRef"=w128) -> ("Motor Values"=w117:dbl[])  [unwired: 1 in, 7 out]
  n272 = call <vilib>:"SD Write Numeric Array.vi"("Numeric Array"=w117, "Name"="Robot Drive Motors") -> ()  [unwired: 8 in, 2 out]
